vi "Example.vi"() -> ()   [LabVIEW 2019, in "Tiles.lvlib"]
uses:
  Tiles.lvlib
  <vilib>/Platform/TimedLoop/XDataNode/timing_clust.ctl
  <vilib>/Platform/TimedLoop/XDataNode/nitl_modes.ctl
  <vilib>/Platform/TimedLoop/XDataNode/wakeup.ctl
  <vilib>/rvi/Emulation/niFpgaGetClockAttributes.vi
  <vilib>/rvi/Emulation/niFpgaSctlEmulationGetInTimedLoop.vi
  <vilib>/rvi/Emulation/niFpgaEmulationReportErrorSimple.vi
  <vilib>/rvi/Emulation/niFpgaCriticalErrorInLSC.vi
  <vilib>/rvi/Memory/Memory_Emulation/nirvimemoryFastEmulation.vi
  <vilib>/rvi/Memory/Memory_Emulation/nirvimemoryEmulation.vi
  <vilib>/rvi/Emulation/niFpgaEmulationIsFPGAContextNoSignature.vi
  <vilib>/rvi/DataTransferAndStorage/Container/Common/niFpgaContainerGetUniqueNameForEmu.vi
  <vilib>/rvi/Emulation/niFpgaProcessEmulError.vi
  <vilib>/rvi/errors/nirviReportUnexpectedCaseInternalError (U32).vi
  <vilib>/platform/TimedLoop/XDataNode/XDataNode.xnode
  <vilib>/rvi/DataTransferAndStorage/Container/XNode/niFpgaContainer.xnode
  <vilib>/Platform/TimedLoop/XDataNode/XDNodeRunTimeDep.lvlib
  Shared/Shared.lvlib
  VGA/VGA.lvlib
panel:
  in  "ReplaceColor":fxp<+,3,3>
  in  "ColorToReplace":fxp<+,3,3>
  in  "Background":fxp<+,3,3>
  in  "Rotate":u8
  in  "TileNo":u8=2
  in  "y":u16
  in  "x":u16
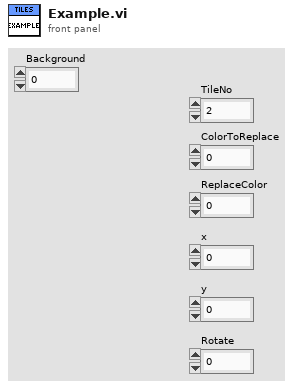
[diagram p1: front panel]
types:
  T1 = typedef "XDNodeRunTimeDep.lvlib/timing_clust.ctl" = cluster{"Expected End [f-1]":u64, "Actual End [f-1]":u64, "Finished Late? [f-1]":bool, "Expected End [i-1]":u64, "Actual End [i-1]":u64, "Finished Late? [i-1]":bool, "Expected Start [i]":u64, "Actual Start [i]":u64, "Expected Start [f]":u64, "Actual Start [f]":u64, "Source Name":string, "Structure Name":string, "Period":i64, "Deadline":i64, "Offset":i64, "Start":i64, "Priority":i32, "Timeout":i32, "Mode":T2, "Wakeup Reason":T3, "Error":errorcluster, "Source Type":string, "Secondary Source Type":string, "Global End Time":u64, "Global Start Time":u64, "Frame Duration":u64, "Iteration Duration":u64, "Assigned CPU":i32, "I/O Scan Engine Mode":u32}
  T2 = typedef "XDNodeRunTimeDep.lvlib/nitl_modes.ctl" = enum32{"No Change", "Process missed periods, maintain original phase", "Discard missed periods, maintain original phase", "Process missed periods, ignore original phase", "Discard missed periods, ignore original phase"}
  T3 = typedef "XDNodeRunTimeDep.lvlib/wakeup.ctl" = enum32{"Normal", "Aborted", "Asynchronous wakeup", "Timing source error", "Timed loop error", "Timeout"}
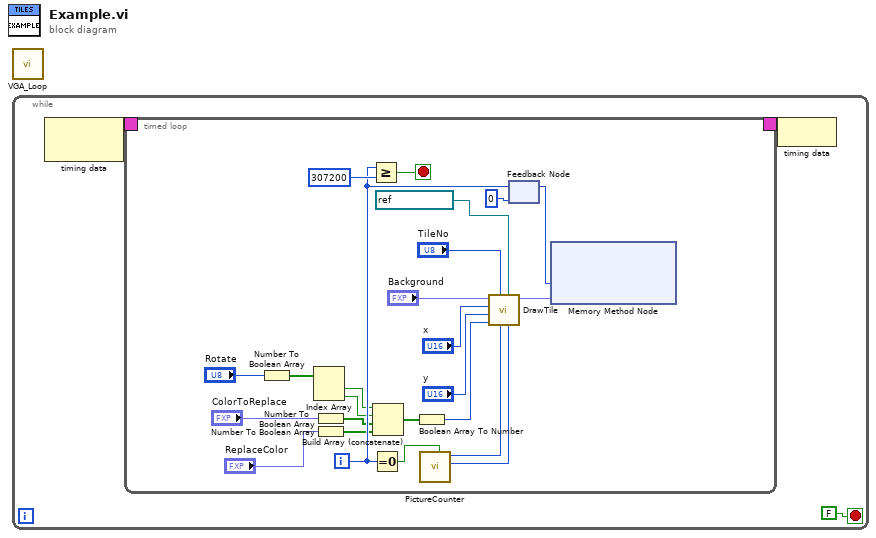
[diagram p0: block diagram]
diagram:
  n1 = call "VGA_Loop.vi"() -> ()  [unwired: 12 in]
  n2 = while {
    stop <- FALSE stop-if-true
    n3 = node-c288() -> (w3:T1)  [unwired: 1 in]
    n4 = timed-loop {
      timing: w3 -> [_]
      timing-out: [_] -> w2
      i -> [w17]
      stop <- w26 stop-if-true
      n5 = Number To Boolean Array(number="Rotate") -> (Boolean array=w12:bool[])
      n6 = Index Array(array=w12) -> (element #1=w11:bool, element #2=w10:bool)  [unwired: 2 in]
      n7 = Number To Boolean Array(number="ColorToReplace") -> (Boolean array=w9:bool[])
      n8 = Number To Boolean Array(number="ReplaceColor") -> (Boolean array=w8:bool[])
      n9 = Greater Or Equal?(x=w17, y=307200) -> (x >= y?=w26:bool)
      n10 = Equal To 0?(x=w17) -> (x = 0?=w16:bool)
      n11 = Build Array (concatenate)(w11, w10, w9, w8) -> (w7:bool[])
      n12 = Boolean Array To Number(Boolean array=w7) -> (number=w4:u8)
      n13 = call "PictureCounter.vi"("Reset? (f)"=w16) -> ("y"=w21:u16, "x"=w22:u16)  [unwired: 9 in]
      n14 = call "DrawTile.vi"("index_y"=w21, "Tilebuffer"=refnum<k21> "TileBuffer", "index_x"=w22, "TileNo"="TileNo", "Modifier"=w4, "pos_y"="y", "pos_x"="x", "color_in"="Background") -> ("color_out"=w25:fxp<+,3,3>)  [unwired: 3 in]
      n15 = feedback-in #1(w17) -> ()
      n16 = feedback #1(0) -> (w19:i32)
      n17 = xnode ("Memory Method Node")("Address"=w19, "Data"=w25) -> ()  [unwired: 1 in, 1 out]
    }
    n18 = node-c288(w2) -> ()
  }
